vi "Countdown.vi"(0 "Min":u32, 5 "sec":u32, 11 "error in (no error)":errorcluster caption="Fehler (Eingang, kein Fehler)", 13 "Aktion":enum16{"init", "prüfen", "löschen"}(ring)) -> (4 "Countdown Anzeige":dbl format="%<%M:%S>T", 6 "Laufleiste":dbl, 8 "Zeit abgelaufen":bool, 10 "Laufleistenbereich":u32, 15 "error out":errorcluster caption="Fehler (Ausgang)")   [LabVIEW 2020, in "EPA 1065.lvlib" / "Chiller NO2 1065-376.lvlib"]
uses:
  EPA 1065/Chiller NO2 1065-376/Chiller NO2 1065-376.lvlib
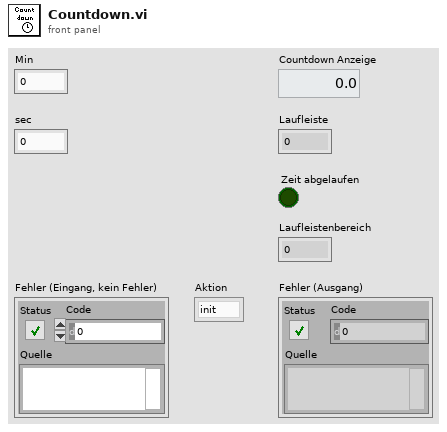
[diagram p1: front panel]
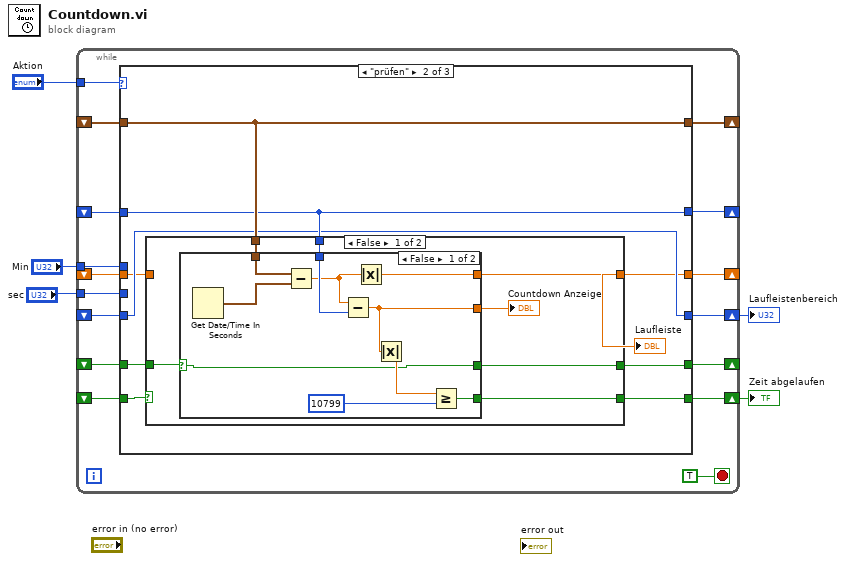
[diagram p0: block diagram]
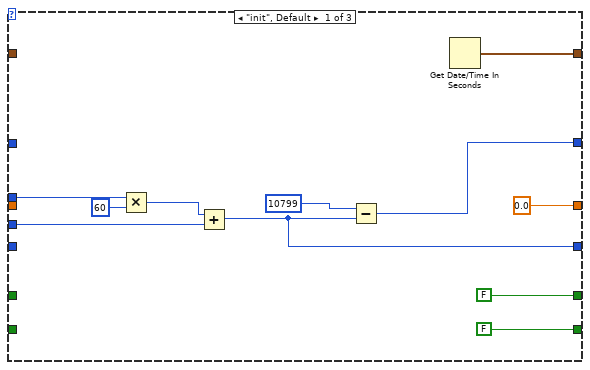
[diagram p2: hidden frame]
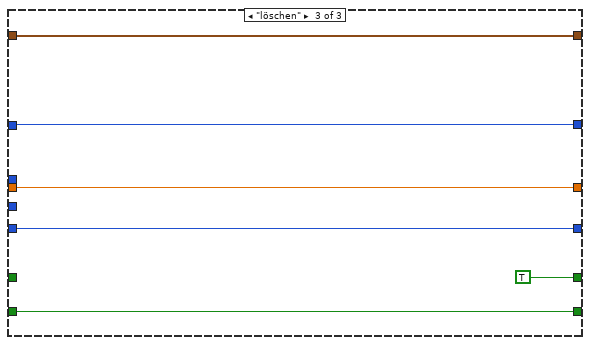
[diagram p5: hidden frame]
diagram:
  n1 = while {
    shift-right: [w20] -> _
    shift-left: _ -> [w19]
    tunnel: "Min" -> [w18]
    tunnel: "sec" -> [w17]
    shift-right: [w16] -> _
    shift-left: _ -> [w15]
    tunnel: "Aktion" -> [w14]
    shift-right: [w13] -> w2
    shift-left: _ -> [w12]
    shift-right: [w11] -> w1
    shift-left: _ -> [w10]
    shift-right: [w9] -> _
    shift-left: _ -> [w8]
    shift-right: [w7] -> _
    shift-left: _ -> [w6]
    stop <- TRUE stop-if-true
    n2 = case shown="\"prüfen\"" w14 {
      tunnel: [w32 w41 w64] -> w20
      tunnel: w19 -> [_ w41 w64]
      tunnel: w18 -> [w31 _ _]
      tunnel: w17 -> [w28 _ _]
      tunnel: [w26 w40 w65] -> w16
      tunnel: w15 -> [_ w40 w65]
      tunnel: [FALSE w39 w66] -> w13
      tunnel: w12 -> [_ w38 w66]
      tunnel: [w24 w37 w63] -> w11
      tunnel: w10 -> [_ w37 w63]
      tunnel: [0.0 w36 w68] -> w9
      tunnel: w8 -> [_ w35 w68]
      tunnel: [FALSE w33 TRUE] -> w7
      tunnel: w6 -> [_ w34 _]
      frame "init", Default {
        n3 = Multiply(x=w31, y=u32 60) -> (x*y=w29:u32)
        n4 = Add(x=w29, y=w28) -> (x+y=w24:u32)
        n5 = Subtract(x=u32 10799 ("y"), y=w24) -> (x-y=w26:u32)
        n6 = Get Date/Time In Seconds() -> (seconds since 1Jan1904=w32:timestamp)
      }
      frame "prüfen" {
        n7 = case shown="False" w38 {
          selector: w38 -> [_ w62]
          tunnel: w41 -> [w48 _]
          tunnel: w40 -> [w47 _]
          tunnel: [w45 w62] -> w39
          tunnel: [w44 w61] -> w36
          tunnel: w35 -> [_ w61]
          tunnel: w34 -> [w43 w60]
          tunnel: [w42 w60] -> w33
          frame False {
            n8 = case shown="False" w43 {
              selector: w43 -> [w49 w59]
              tunnel: w48 -> [w57 _]
              tunnel: w47 -> [w56 _]
              tunnel: [w55 _] -> w46
              tunnel: [w53 _] -> w45
              tunnel: [w50 _] -> w44
              tunnel: [w49 w59] -> w42
              frame False {
                n9 = Get Date/Time In Seconds() -> (seconds since 1Jan1904=w58:timestamp)
                n10 = Subtract(x=w57, y=w58) -> (x-y=w51:dbl)
                n11 = Subtract(x=w51, y=w56) -> (x-y=w55:dbl)
                n12 = Absolute Value(x=w51) -> (abs(x)=w50:dbl)
                n13 = Absolute Value(x=w55) -> (abs(x)=w54:dbl)
                n14 = Greater Or Equal?(x=w54, y=u32 10799) -> (x >= y?=w53:bool)
              }
              frame True {
              }
            }
            "Countdown Anzeige" <- w46
          }
          frame True {
          }
        }
        "Laufleiste" <- w36
      }
      frame "löschen" {
      }
    }
  }
  "Zeit abgelaufen" <- w2
  "Laufleistenbereich" <- w1
